vi "FGV_HovaCAL_Interface_AutoLin_MFC.vi"(6 "Aktion":T1, 8 "error in (no error)":errorcluster caption="Fehler (Eingang, kein Fehler)", 10 "MFV Komponente fix":u16[](array[numeric]), 11 "AutoLin MFC":u16(ring) items=["MFV0", "MFV1", "MFV2"]) -> (0 "error out":errorcluster caption="Fehler (Ausgang)", 1 "fix conf":bool, 2 "MFV Komponente fix out":u16[](array[numeric]), 3 "AutoLin MFC out":u16)   [LabVIEW 2020, in "Linearisierung v2.lvlib" / "Gasteiler.lvlib" / "HovaCAL_Interface.lvlib" / "Kommunikation.lvlib"]
uses:
  Kommunikation.lvlib
  Aktion FGV HovaCAL Interface Autolin.ctl
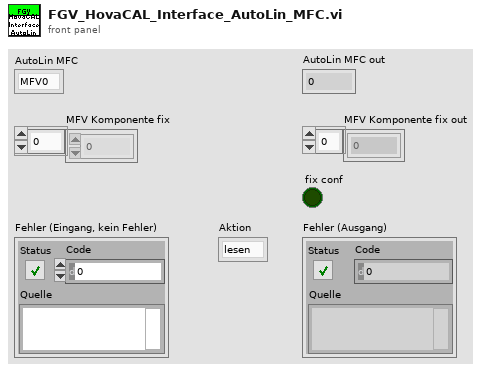
[diagram p1: front panel]
types:
  T1 = typedef "Linearisierung v2.lvlib/Gasteiler.lvlib/HovaCAL_Interface.lvlib/Kommunikation.lvlib/Aktion FGV HovaCAL Interface Autolin.ctl" = enum16{"lesen", "schreiben", "MFC Komponente fix setzen", "init"}
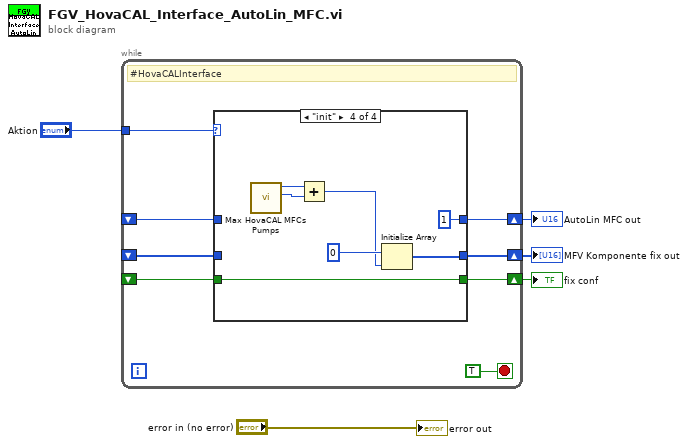
[diagram p0: block diagram]
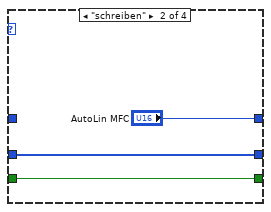
[diagram p3: hidden frame]
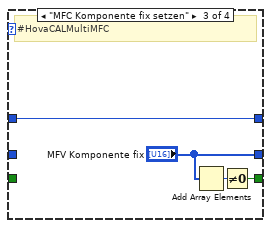
[diagram p4: hidden frame]
diagram:
  n1 = while {
    tunnel: "Aktion" -> [w12]
    shift-right: [w11] -> w4
    shift-left: _ -> [w10]
    shift-right: [w9] -> w2
    shift-left: _ -> [w8]
    shift-right: [w7] -> w1
    shift-left: _ -> [w6]
    stop <- TRUE stop-if-true
    # "#HovaCALInterface"
    n2 = case shown="\"init\"" w12 {
      tunnel: [w16 "AutoLin MFC" w23 u16 1 ("AutoLin MFC")] -> w11
      tunnel: w10 -> [w16 _ w23 _]
      tunnel: [w15 w18 "MFV Komponente fix" w24] -> w9
      tunnel: w8 -> [w15 w18 _ _]
      tunnel: [w14 w17 w21 w30] -> w7
      tunnel: w6 -> [w14 w17 _ w30]
      frame "lesen", Default {
      }
      frame "schreiben" {
      }
      frame "MFC Komponente fix setzen" {
        # "#HovaCALMultiMFC"
        n3 = Add Array Elements(numeric array="MFV Komponente fix") -> (sum=w20:u16)
        n4 = Not Equal To 0?(x=w20) -> (x != 0?=w21:bool)
      }
      frame "init" {
        n5 = call "Max HovaCAL MFCs Pumps.vi"() -> ("max Pumps"=w26:i32, "max MFCs"=w27:i32)  [unwired: 10 in]
        n6 = Add(x=w27, y=w26) -> (x+y=w25:i32)
        n7 = Initialize Array(u16 0 ("AutoLin MFC"), w25) -> (w24:u16[])
      }
    }
  }
  "AutoLin MFC out" <- w4
  "MFV Komponente fix out" <- w2
  "fix conf" <- w1
  "error out" <- "error in (no error)"
